vi "aplicatie bd.vi"() -> ()   [LabVIEW 2022 SP3]
uses:
  <vilib>/addons/database/Connection.llb/DB Tools Open Connec (Path).vi
  <vilib>/addons/database/NI_Database_API.lvlib
panel:
  in  "Home Button":bool
  in  "Check":bool
  in  "Parola":string
  out "Array 3":string[](array[string])
  in  "Nume profesor":string
  in  "Search Button 2":bool
  in  "Back 2":bool
  out "Array 2":string[](array[string])
  in  "Stop Button":bool
  in  "Search Button":bool
  in  "Nume student":string
  in  "Back 1":bool
  in  "Profesor":bool
  in  "Student":bool
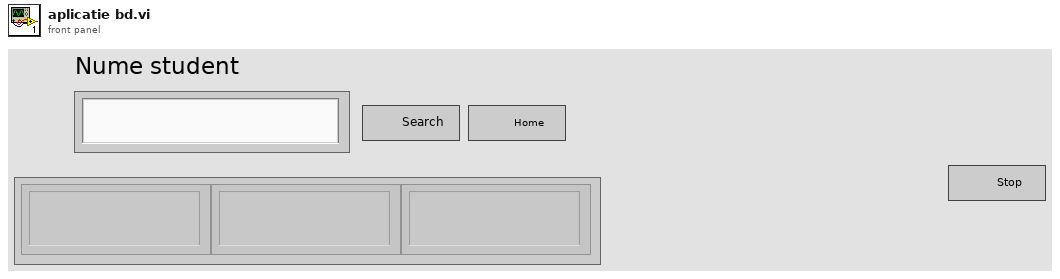
[diagram p1: front panel]
types:
  T1 = typedef "NI_Database_API.lvlib/Conn ObjectReference.ctl" = refnum<k1>
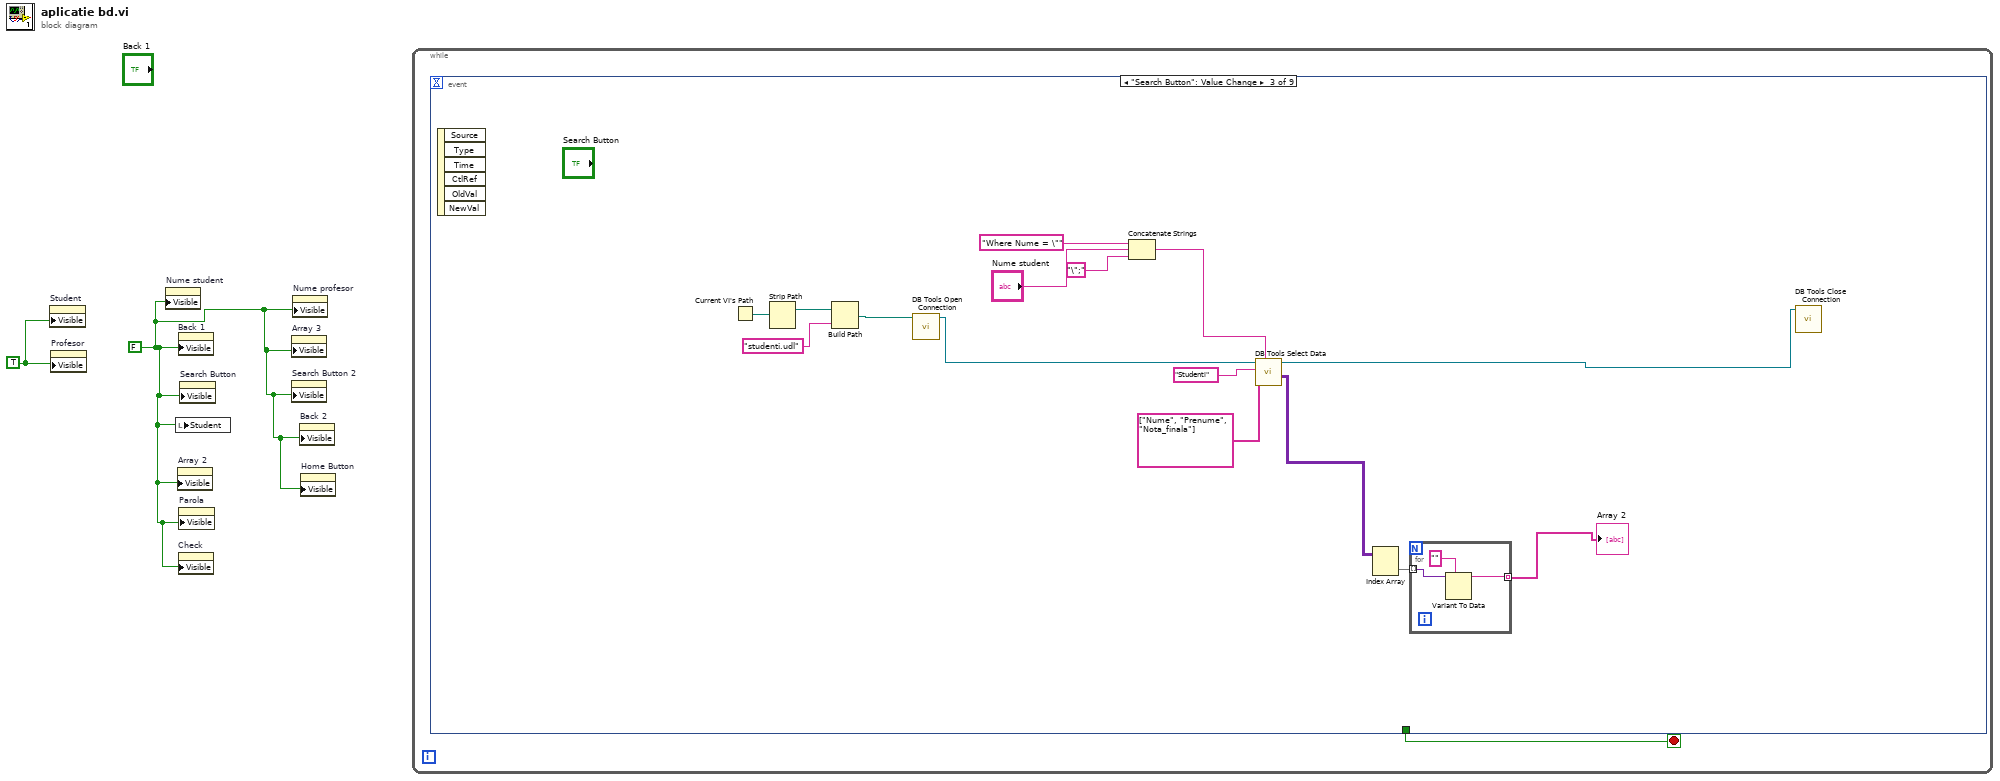
[diagram p0: block diagram]
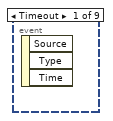
[diagram p2: hidden frame]
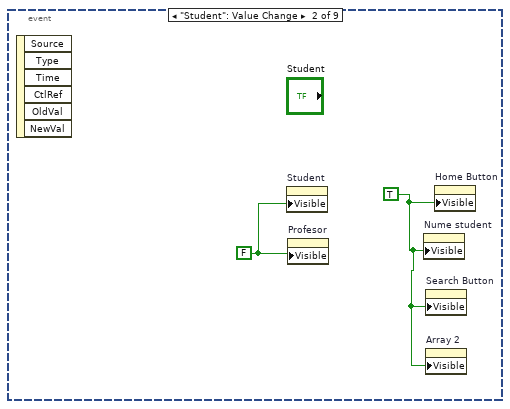
[diagram p3: hidden frame]
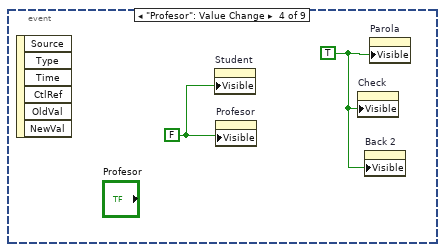
[diagram p4: hidden frame]
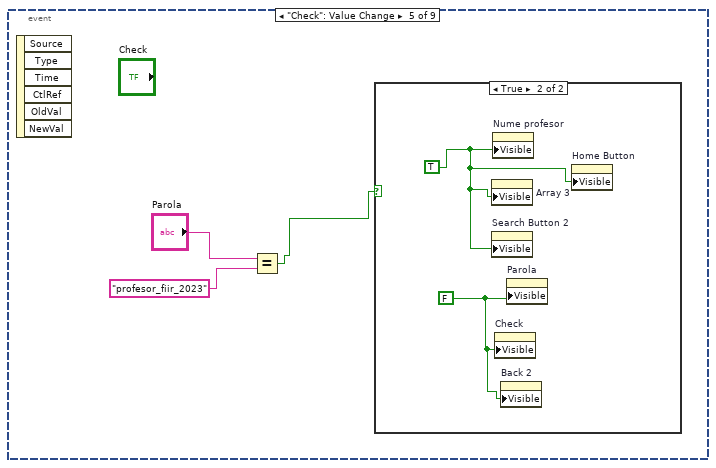
[diagram p5: hidden frame]
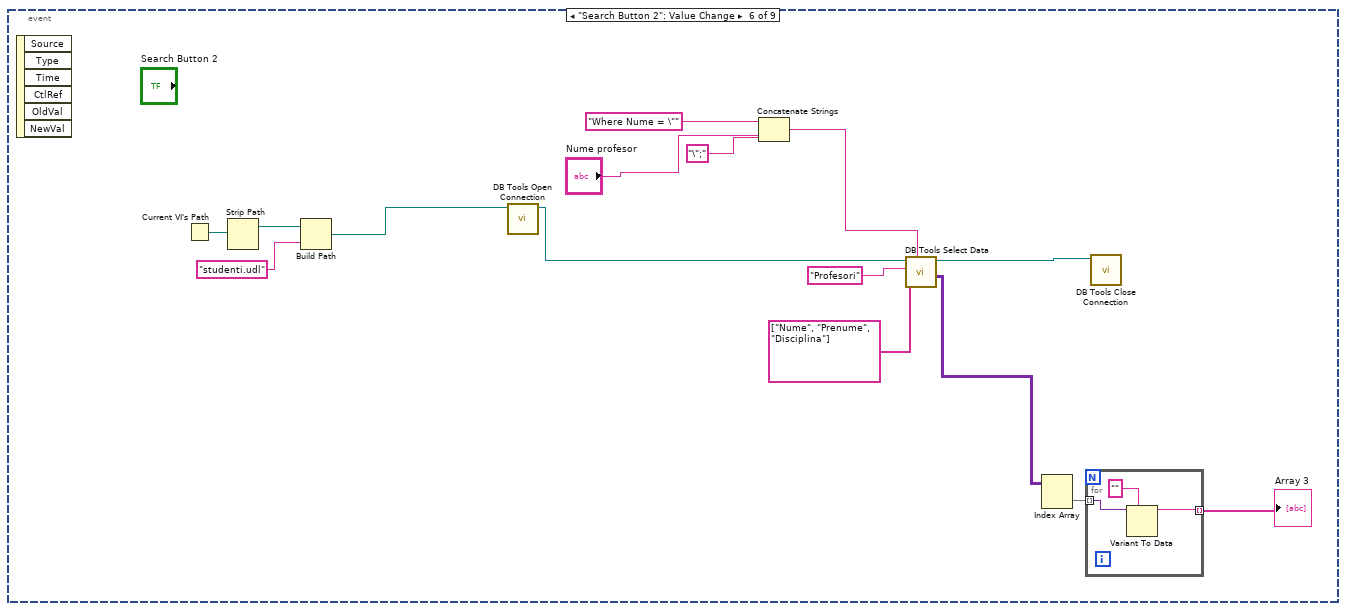
[diagram p7: hidden frame]
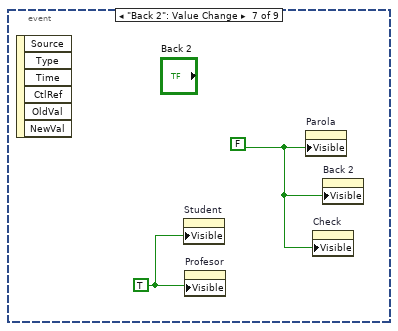
[diagram p8: hidden frame]
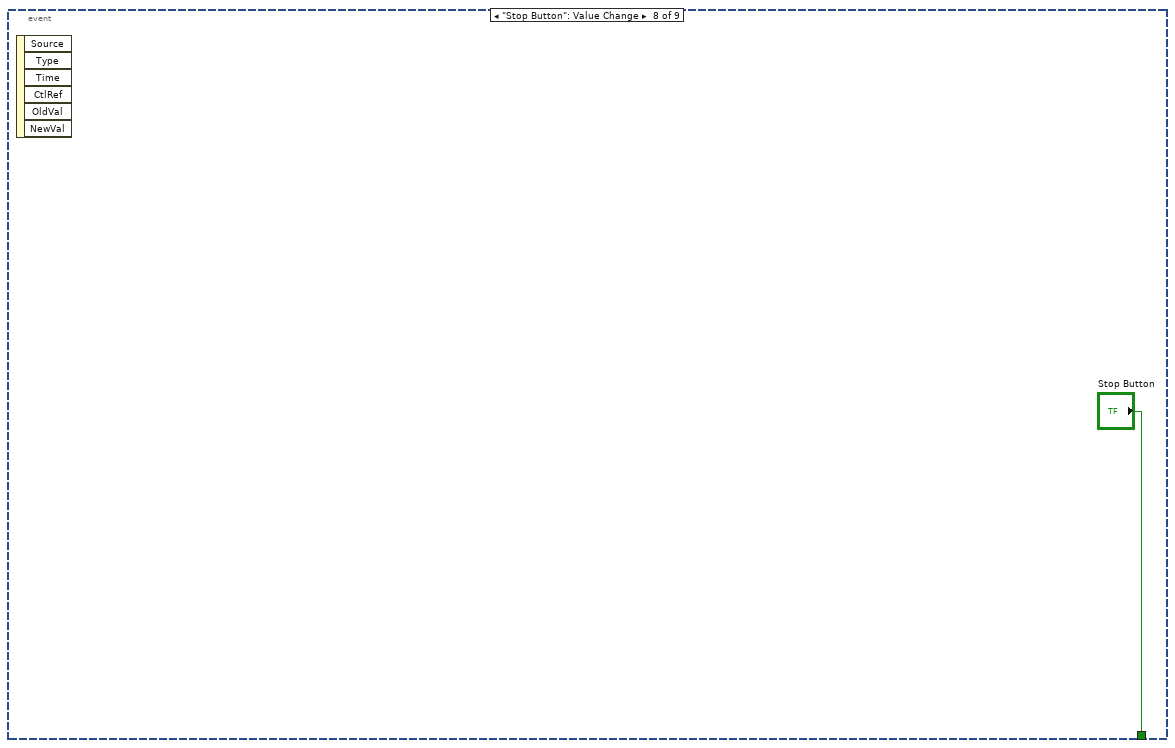
[diagram p9: hidden frame]
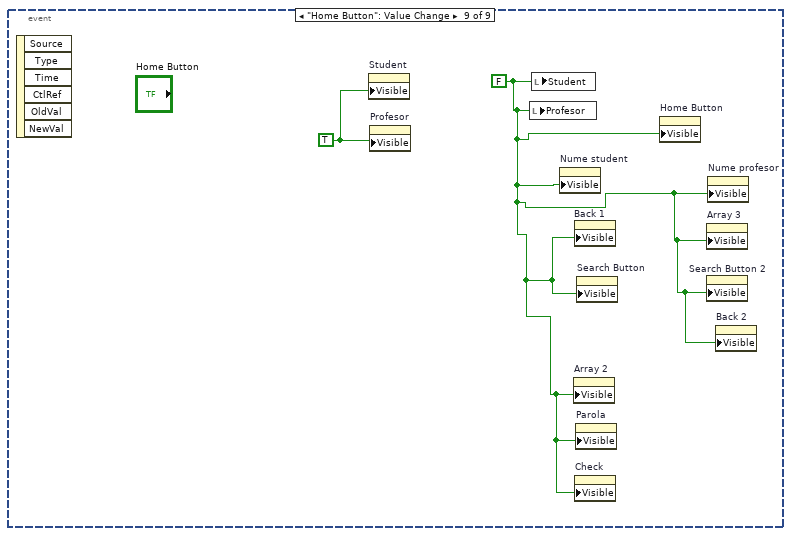
[diagram p10: hidden frame]
diagram:
  w2 = TRUE ("Visible")
  w1 = FALSE ("Visible")
  n1 = property on="Student" class="Bool (strict)"("Visible"=w2) -> ()  [unwired: 2 in, 2 out]
  n2 = property on="Profesor" class="Bool (strict)"("Visible"=w2) -> ()  [unwired: 2 in, 2 out]
  n3 = property on="Nume student" class="Str"("Visible"=w1) -> ()  [unwired: 2 in, 2 out]
  n4 = local write "Student"(w1) -> ()
  n5 = property on="Array 2" class="Arr (strict)"("Visible"=w1) -> ()  [unwired: 2 in, 2 out]
  n6 = property on="Back 1" class="Bool (strict)"("Visible"=w1) -> ()  [unwired: 2 in, 2 out]
  n7 = property on="Check" class="Bool (strict)"("Visible"=w1) -> ()  [unwired: 2 in, 2 out]
  n8 = property on="Parola" class="Str"("Visible"=w1) -> ()  [unwired: 2 in, 2 out]
  n9 = property on="Search Button" class="Bool"("Visible"=w1) -> ()  [unwired: 2 in, 2 out]
  n10 = property on="Array 3" class="Arr (strict)"("Visible"=w1) -> ()  [unwired: 2 in, 2 out]
  n11 = property on="Search Button 2" class="Bool"("Visible"=w1) -> ()  [unwired: 2 in, 2 out]
  n12 = property on="Nume profesor" class="Str"("Visible"=w1) -> ()  [unwired: 2 in, 2 out]
  n13 = property on="Back 2" class="Bool (strict)"("Visible"=w1) -> ()  [unwired: 2 in, 2 out]
  n14 = property on="Home Button" class="Bool (strict)"("Visible"=w1) -> ()  [unwired: 2 in, 2 out]
  n15 = while {
    stop <- w3 stop-if-true
    n16 = event shown="[2] \"Search Button\": Value Change" {
      selector: _ -> [_ _ _ _ _ _ _ _ _]
      dyn-events: _ -> [_ _ _ _ _ _ _ _ _]
      timeout: _ -> [_ _ _ _ _ _ _ _ _]
      tunnel: [_ _ _ _ _ _ _ "Stop Button" _] -> w3
      event Timeout {
        n17 = event-data() -> ()  [unwired: 1 in, 3 out]
      }
      event "Student": Value Change {
        w4 = TRUE ("Visible")
        w5 = FALSE ("Visible")
        n18 = event-data() -> ()  [unwired: 1 in, 6 out]
        n19 = property on="Student" class="Bool (strict)"("Visible"=w5) -> ()  [unwired: 2 in, 2 out]
        n20 = property on="Profesor" class="Bool (strict)"("Visible"=w5) -> ()  [unwired: 2 in, 2 out]
        n21 = property on="Nume student" class="Str"("Visible"=w4) -> ()  [unwired: 2 in, 2 out]
        n22 = property on="Search Button" class="Bool"("Visible"=w4) -> ()  [unwired: 2 in, 2 out]
        n23 = property on="Array 2" class="Arr (strict)"("Visible"=w4) -> ()  [unwired: 2 in, 2 out]
        n24 = property on="Home Button" class="Bool (strict)"("Visible"=w4) -> ()  [unwired: 2 in, 2 out]
      }
      event "Search Button": Value Change {
        n25 = event-data() -> ()  [unwired: 1 in, 6 out]
        n26 = Current VI's Path() -> (path=w9:path)
        n27 = Strip Path(path=w9) -> (stripped path=w8:path)  [unwired: 1 out]
        n28 = Build Path(base path=w8, name or relative path="studenti.udl" ("string")) -> (appended path=w6:path)
        n29 = call-poly <vilib>:"DB Tools Open Connection.vi"("connection information"=w6) -> ("connection reference"=w18:T1)  [unwired: 7 in, 1 out]
        n30 = Concatenate Strings("Where Nume = \"" ("string"), "Nume student", "\";" ("string")) -> (w11:string)
        n31 = call <vilib>:"DB Tools Select Data.vi"("condition"=w11, "columns"=string[] ["Nume", "Prenume", "Nota_finala"], "table"="Studenti", "connection reference"=w18) -> ("data"=w16:variant[][], "connection reference out"=w15:T1)  [unwired: 2 in, 1 out]
        n32 = Index Array(array=w16) -> (element=w17:variant[])  [unwired: 2 in]
        n33 = for {
          tunnel: w17 -> [w23] mode=indexing
          tunnel: [w22] -> w10 mode=indexing
          n34 = Variant To Data(type="", Variant=w23) -> (data=w22:string)  [unwired: 1 in, 1 out]
        }
        "Array 2" <- w10
        n35 = call <vilib>:"DB Tools Close Connection.vi"("connection reference"=w15) -> ()  [unwired: 6 in, 1 out]
      }
      event "Profesor": Value Change {
        w24 = TRUE ("Visible")
        w25 = FALSE ("Visible")
        n36 = event-data() -> ()  [unwired: 1 in, 6 out]
        n37 = property on="Student" class="Bool (strict)"("Visible"=w25) -> ()  [unwired: 2 in, 2 out]
        n38 = property on="Profesor" class="Bool (strict)"("Visible"=w25) -> ()  [unwired: 2 in, 2 out]
        n39 = property on="Check" class="Bool (strict)"("Visible"=w24) -> ()  [unwired: 2 in, 2 out]
        n40 = property on="Back 2" class="Bool (strict)"("Visible"=w24) -> ()  [unwired: 2 in, 2 out]
        n41 = property on="Parola" class="Str"("Visible"=w24) -> ()  [unwired: 2 in, 2 out]
      }
      event "Check": Value Change {
        n42 = event-data() -> ()  [unwired: 1 in, 6 out]
        n43 = Equal?(x="Parola", y="profesor_fiir_2023") -> (x = y?=w26:bool)
        n44 = case shown="True" w26 {
          frame False {
          }
          frame True {
            w30 = FALSE ("y")
            w29 = TRUE ("y")
            n45 = property on="Array 3" class="Arr (strict)"("Visible"=w29) -> ()  [unwired: 2 in, 2 out]
            n46 = property on="Search Button 2" class="Bool"("Visible"=w29) -> ()  [unwired: 2 in, 2 out]
            n47 = property on="Nume profesor" class="Str"("Visible"=w29) -> ()  [unwired: 2 in, 2 out]
            n48 = property on="Check" class="Bool (strict)"("Visible"=w30) -> ()  [unwired: 2 in, 2 out]
            n49 = property on="Back 2" class="Bool (strict)"("Visible"=w30) -> ()  [unwired: 2 in, 2 out]
            n50 = property on="Parola" class="Str"("Visible"=w30) -> ()  [unwired: 2 in, 2 out]
            n51 = property on="Home Button" class="Bool (strict)"("Visible"=w29) -> ()  [unwired: 2 in, 2 out]
          }
        }
      }
      event "Search Button 2": Value Change {
        n52 = event-data() -> ()  [unwired: 1 in, 6 out]
        n53 = Current VI's Path() -> (path=w34:path)
        n54 = Strip Path(path=w34) -> (stripped path=w33:path)  [unwired: 1 out]
        n55 = Build Path(base path=w33, name or relative path="studenti.udl" ("string")) -> (appended path=w31:path)
        n56 = call-poly <vilib>:"DB Tools Open Connection.vi"("connection information"=w31) -> ("connection reference"=w43:T1)  [unwired: 7 in, 1 out]
        n57 = Concatenate Strings("Where Nume = \"" ("string"), "Nume profesor", "\";" ("string")) -> (w38:string)
        n58 = call <vilib>:"DB Tools Select Data.vi"("condition"=w38, "columns"=string[] ["Nume", "Prenume", "Disciplina"], "table"="Profesori", "connection reference"=w43) -> ("data"=w41:variant[][], "connection reference out"=w35:T1)  [unwired: 2 in, 1 out]
        n59 = Index Array(array=w41) -> (element=w42:variant[])  [unwired: 2 in]
        n60 = for {
          tunnel: w42 -> [w48] mode=indexing
          tunnel: [w47] -> w37 mode=indexing
          n61 = Variant To Data(type="", Variant=w48) -> (data=w47:string)  [unwired: 1 in, 1 out]
        }
        "Array 3" <- w37
        n62 = call <vilib>:"DB Tools Close Connection.vi"("connection reference"=w35) -> ()  [unwired: 6 in, 1 out]
      }
      event "Back 2": Value Change {
        w50 = TRUE ("Visible")
        w49 = FALSE ("Visible")
        n63 = event-data() -> ()  [unwired: 1 in, 6 out]
        n64 = property on="Student" class="Bool (strict)"("Visible"=w50) -> ()  [unwired: 2 in, 2 out]
        n65 = property on="Profesor" class="Bool (strict)"("Visible"=w50) -> ()  [unwired: 2 in, 2 out]
        n66 = property on="Parola" class="Str"("Visible"=w49) -> ()  [unwired: 2 in, 2 out]
        n67 = property on="Check" class="Bool (strict)"("Visible"=w49) -> ()  [unwired: 2 in, 2 out]
        n68 = property on="Back 2" class="Bool (strict)"("Visible"=w49) -> ()  [unwired: 2 in, 2 out]
      }
      event "Stop Button": Value Change {
        n69 = event-data() -> ()  [unwired: 1 in, 6 out]
      }
      event "Home Button": Value Change {
        w52 = FALSE ("Student")
        w53 = TRUE ("Visible")
        n70 = event-data() -> ()  [unwired: 1 in, 6 out]
        n71 = property on="Student" class="Bool (strict)"("Visible"=w53) -> ()  [unwired: 2 in, 2 out]
        n72 = property on="Profesor" class="Bool (strict)"("Visible"=w53) -> ()  [unwired: 2 in, 2 out]
        n73 = local write "Profesor"(w52) -> ()
        n74 = local write "Student"(w52) -> ()
        n75 = property on="Nume student" class="Str"("Visible"=w52) -> ()  [unwired: 2 in, 2 out]
        n76 = property on="Array 2" class="Arr (strict)"("Visible"=w52) -> ()  [unwired: 2 in, 2 out]
        n77 = property on="Back 1" class="Bool (strict)"("Visible"=w52) -> ()  [unwired: 2 in, 2 out]
        n78 = property on="Check" class="Bool (strict)"("Visible"=w52) -> ()  [unwired: 2 in, 2 out]
        n79 = property on="Parola" class="Str"("Visible"=w52) -> ()  [unwired: 2 in, 2 out]
        n80 = property on="Search Button" class="Bool"("Visible"=w52) -> ()  [unwired: 2 in, 2 out]
        n81 = property on="Home Button" class="Bool (strict)"("Visible"=w52) -> ()  [unwired: 2 in, 2 out]
        n82 = property on="Array 3" class="Arr (strict)"("Visible"=w52) -> ()  [unwired: 2 in, 2 out]
        n83 = property on="Search Button 2" class="Bool"("Visible"=w52) -> ()  [unwired: 2 in, 2 out]
        n84 = property on="Nume profesor" class="Str"("Visible"=w52) -> ()  [unwired: 2 in, 2 out]
        n85 = property on="Back 2" class="Bool (strict)"("Visible"=w52) -> ()  [unwired: 2 in, 2 out]
      }
    }
  }
